vi "ProjectOpen.vi"(6 "Visible?":bool, 7 "Sequence Context":refnum<k7>, 8 "password":string, 9 "username":string, 10 "Project File Path":path, 11 "Gateway IP Address (\"\": localhost)":string) -> (0 "error out":errorcluster)   [LabVIEW 2015, in "MiscHelperVIs.lvlib"]
uses:
  MiscHelperVIs.lvlib
  controls/VeriStand dotNet References.ctl
  NationalInstruments.VeriStand.ClientAPI
  <vilib>/NI Veristand/Execution/Project/NI_VS Project ExecutionAPI.lvlib
panel:
  in  "error in (no error)":errorcluster
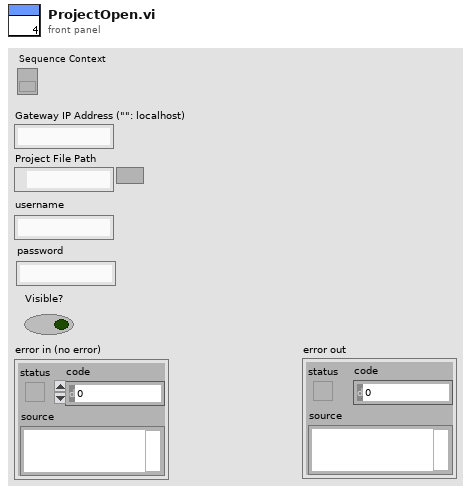
[diagram p1: front panel]
types:
  T1 = typedef "MiscHelperVIs.lvlib/VeriStand dotNet References.ctl" = cluster{"VS Project .NET Refnum":refnum<k24>, "Workspace Manager .NET Refnum":refnum<k24>}
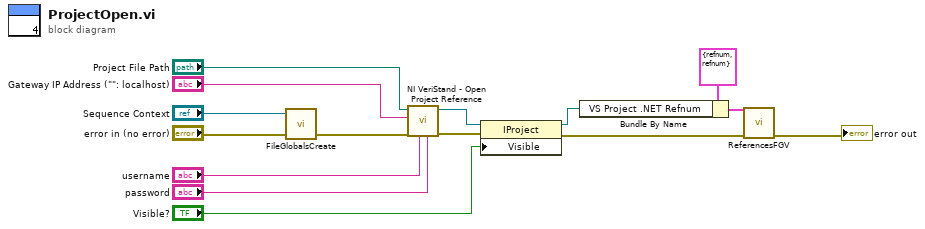
[diagram p0: block diagram]
diagram:
  n1 = call "FileGlobalsCreate.vi"("error in (no error)"="error in (no error)", "Sequence Context"="Sequence Context") -> ("error out"=w9:errorcluster)  [unwired: 3 in]
  n2 = call <vilib>:"NI VeriStand - Open Project Reference.vi"("Password"="password", "Username"="username", "error in (no error)"=w9, "Gateway IP Address (\"\": localhost)"="Gateway IP Address (\"\": localhost)", "Project File Path"="Project File Path") -> ("error out"=w7:errorcluster, "Project Ref"=w8:refnum<k24>)  [unwired: 5 in]
  n3 = property class="IProject"(reference=w8, error in=w7, "Visible"="Visible?") -> (reference out=w2:refnum<k24>, error out=w3:errorcluster)
  n4 = Bundle By Name(cluster=T1 {"VS Project .NET Refnum"=refnum, "Workspace Manager .NET Refnum"=refnum} ("VeriStand dotNET Refs"), "VS Project .NET Refnum"=w2) -> (w5:T1)
  n5 = call "ReferencesFGV.vi"("error in (no error)"=w3, "VeriStand dotNET Refs"=w5) -> ("error out"=→"error out":errorcluster)  [unwired: 8 in, 1 out]
